vi "input image output roi rect.vi"(11 "Refnum in":T1) -> (1 "selected rectangle":i32[](array[numeric]), 3 "Refnum out":T1)   [LabVIEW 2011]
uses:
  <vilib>/vision/Image Controls.llb/IMAQ Image.ctl
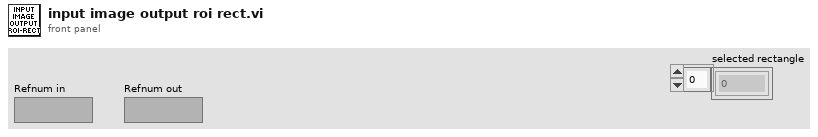
[diagram p1: front panel]
types:
  T1 = typedef "IMAQ Image.ctl" = refnum<image>
  T2 = typedef "IMAQ Rectangle" = cluster{"Left":i32, "Top":i32, "Right":i32, "Bottom":i32, "Rotation":dbl}
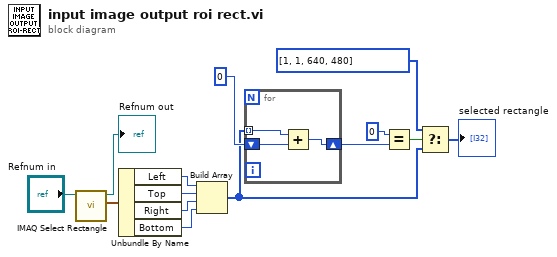
[diagram p0: block diagram]
diagram:
  n1 = call "IMAQ Select Rectangle"("Image In"="Refnum in") -> ("Rectangle"=w10:T2, "Image Out (duplicate)"=→"Refnum out":T1)  [unwired: 7 in, 2 out]
  n2 = Unbundle By Name(w10) -> ("Left"=w12:i32, "Top"=w11:i32, "Right"=w13:i32, "Bottom"=w14:i32)
  n3 = Build Array(w12, w11, w13, w14) -> (w3:i32[])
  n4 = for {
    tunnel: w3 -> [w17] mode=indexing
    shift-right: [w16] -> w6
    shift-left: 0 -> [w15]
    n5 = Add(x=w17, y=w15) -> (x+y=w16:i32)
  }
  n6 = Equal?(x=0, y=w6) -> (x = y?=w4:bool)
  n7 = Select(t=i32[] [1, 1, 640, 480] ("appended array"), s=w4, f=w3) -> (s? t:f=→"selected rectangle":i32[])
